vi "Pololu.Mgr - Move to Saved Position.vi"(6 "Ignore Stops":bool, 8 "error in (no error)":errorcluster, 9 "Position Index":i32, 10 "Channel":u8, 11 "PololuCtrl in":refnum<class "PololuCtrl.lvclass">) -> (0 "error out":errorcluster, 1 "Cmd Bytes(Hex)":string, 2 "Position(Deg)":dbl, 3 "PololuCtrl out":refnum<class "PololuCtrl.lvclass">, 4 "Cmd Bytes(Str)":string)   [LabVIEW 2018, in "PololuCtrl.lvclass"]
uses:
  PololuCtrl.lvclass
  PololuCtrl.lvclass/PololuCtrl.ctl
  SubVIs/Pololu.Message Byte Defs.ctl
  Serial Port/Class/SerialPort.lvclass
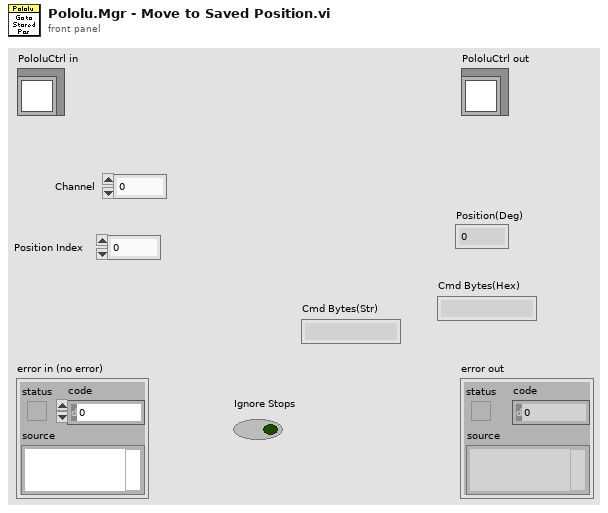
[diagram p1: front panel]
types:
  T1 = typedef "Pololu.Device Config.ctl" = cluster{"Chan":u8, "Accel":u16, "Speed":u16, "Positions":dbl[], "Range Info":T2}
  T2 = typedef "Pololu.Device Range Config.ctl" = cluster{"Min us":dbl, "Max us":dbl, "Min deg":dbl, "Max deg":dbl, "LStopDeg":dbl, "UStopDeg":dbl}
  T3 = cluster{"Channel":u8, "Pos":u16, "Response":u16, "Bytes":u8[], "Query":bool}
  T4 = typedef "Pololu.Message Byte Defs.ctl" = u8
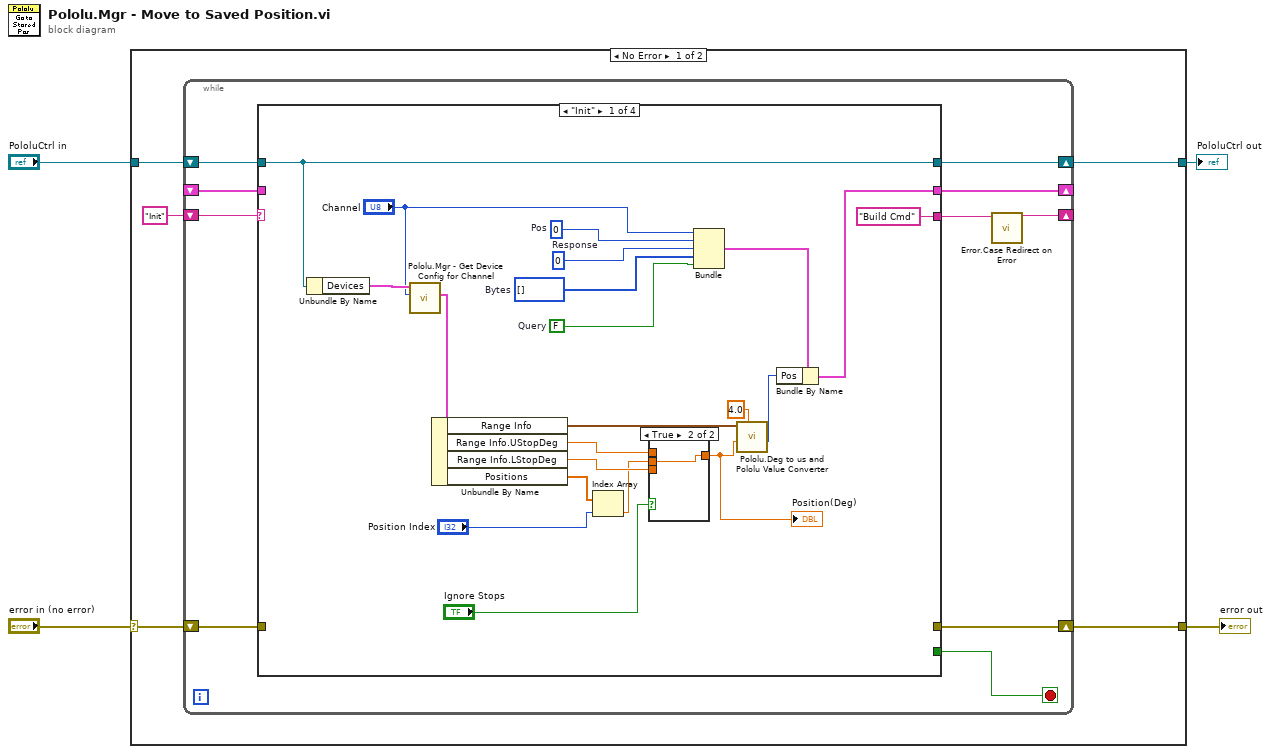
[diagram p0: block diagram]
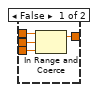
[diagram p2: hidden frame]
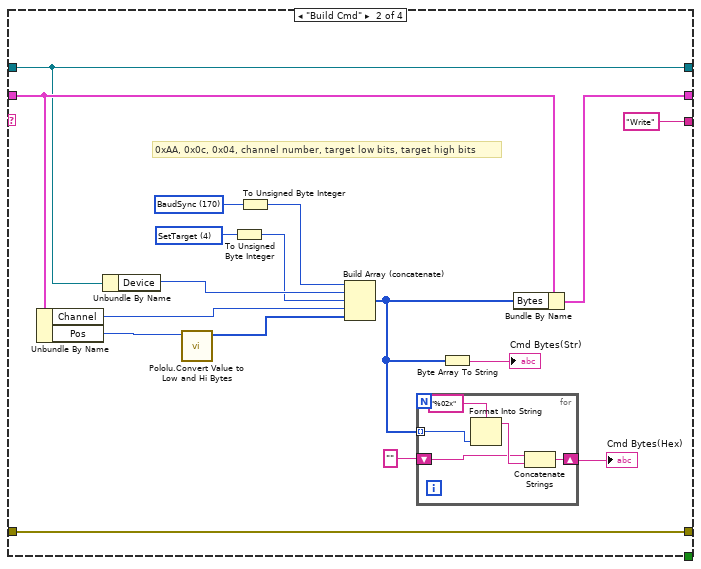
[diagram p3: hidden frame]
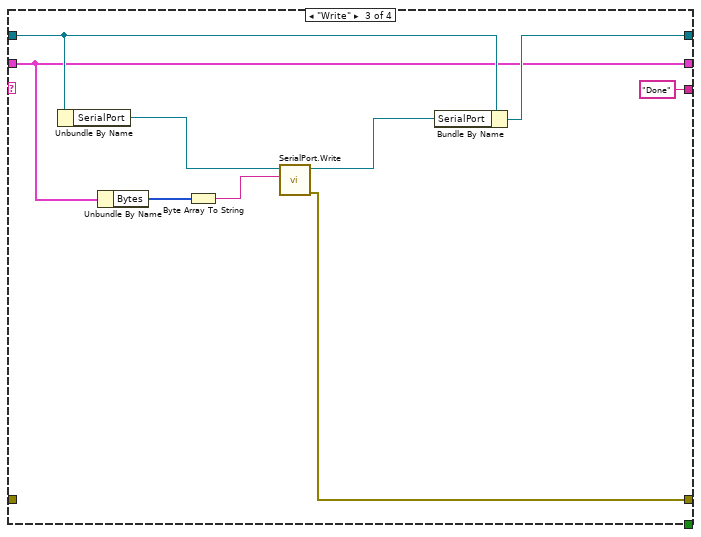
[diagram p4: hidden frame]
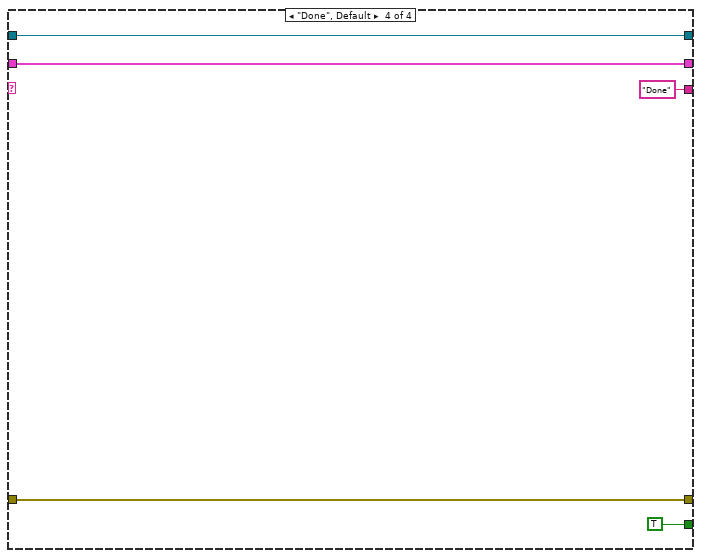
[diagram p5: hidden frame]
diagram:
  n1 = case shown="No Error" "error in (no error)" {
    selector: "error in (no error)" -> [w8 w83]
    tunnel: [w5 w83] -> w3
    tunnel: [w7 w82] -> w1
    tunnel: "PololuCtrl in" -> [w9 w82]
    frame No Error {
      n2 = while {
        shift-right: [w18] -> w7
        shift-left: w9 -> [w19]
        shift-right: [w11] -> w5
        shift-left: w8 -> [w12]
        shift-right: [w15] -> _
        shift-left: "Init" -> [w16]
        shift-right: [w13] -> _
        shift-left: _ -> [w17]
        stop <- w10 stop-if-true
        n3 = case shown="\"Init\"" w16 {
          tunnel: w19 -> [w35 w57 w73 w81]
          tunnel: [w35 w57 w74 w81] -> w18
          tunnel: w17 -> [_ w60 w69 w78]
          tunnel: ["Build Cmd" "Write" "Done" "Done"] -> w14
          tunnel: [w33 w61 w69 w78] -> w13
          tunnel: w12 -> [_ w62 _ w79]
          tunnel: [_ w62 w70 w79] -> w11
          tunnel: [_ _ _ TRUE] -> w10
          frame "Init" {
            w36 = u16 0  # Pos
            w39 = u16 0  # Response
            w37 = FALSE  # Query
            w38 = u8[] []  # Bytes
            n4 = Unbundle By Name(w35) -> ("Devices"=w23:T1[])
            n5 = call "Pololu.Mgr - Get Device Config for Channel.vi"("Channel"="Channel", "Devices"=w23) -> ("Device"=w21:T1)  [unwired: 7 in, 2 out]
            n6 = Unbundle By Name(w21) -> ("Range Info"=w30:T2, "Range Info.UStopDeg"=w32:dbl, "Range Info.LStopDeg"=w31:dbl, "Positions"=w27:dbl[])
            n7 = Index Array(array=w27, index="Position Index") -> (element=w25:dbl)
            n8 = case shown="True" "Ignore Stops" {
              tunnel: w32 -> [w44 _]
              tunnel: w31 -> [w43 _]
              tunnel: w25 -> [w42 w45]
              tunnel: [w41 w45] -> w24
              frame False {
                n9 = In Range and Coerce(upper limit=w44, x=w42, lower limit=w43) -> (coerced(x)=w41:dbl)  [unwired: 1 out]
              }
              frame True {
              }
            }
            "Position(Deg)" <- w24
            n10 = Bundle("Channel"="Channel", "Pos"=w36, "Response"=w39, "Bytes"=w38, "Query"=w37) -> (w34:T3)  [unwired: 1 in]
            n11 = call "Pololu.Deg to us and Pololu Value Converter.vi"("us to Units Mult"=4.0, "Set Pos (Deg)"=w24, "Range Info"=w30) -> ("Cmd units"=w29:u16)  [unwired: 7 in, 1 out]
            n12 = Bundle By Name(cluster=w34, "Pos"=w29) -> (w33:T3)
          }
          frame "Build Cmd" {
            w51 = T4 4 items=["BaudSync"=170, "SetTarget"=4, "Set Speed"=7, "Set Accel"=9, "Get Pos"=16, "Get MovStat"=19, "Get Errors"=33] ("Cmds")
            w52 = T4 170 items=["BaudSync"=170, "SetTarget"=4, "Set Speed"=7, "Set Accel"=9, "Get Pos"=16, "Get MovStat"=19, "Get Errors"=33] ("Cmds")
            # "0xAA, 0x0c, 0x04, channel number, target low bits, target high bits"
            n13 = Unbundle By Name(w60) -> ("Channel"=w59:u8, "Pos"=w58:u16)
            n14 = Unbundle By Name(w57) -> ("Device"=w56:u8)
            n15 = call "Pololu.Convert Value to Low and Hi Bytes.vi"("Value"=w58) -> ("Low_Hi Bytes"=w53:u8[])  [unwired: 10 in]
            n16 = To Unsigned Byte Integer(number=w51) -> (unsigned 8bit integer=w54:T4)
            n17 = To Unsigned Byte Integer(number=w52) -> (unsigned 8bit integer=w55:T4)
            n18 = Build Array (concatenate)(w55, w56, w54, w59, w53) -> (w47:T4[])
            n19 = for {
              tunnel: w47 -> [w67] mode=indexing
              shift-right: [w65] -> w48
              shift-left: "" -> [w63]
              n20 = Format Into String(format string="%02x", w67) -> (resulting string=w64:string)  [unwired: 2 in, 1 out]
              n21 = Concatenate Strings(w63, w64) -> (w65:string)
            }
            "Cmd Bytes(Hex)" <- w48
            n22 = Byte Array To String(unsigned byte array=w47) -> (string=→"Cmd Bytes(Str)":string)
            n23 = Bundle By Name(cluster=w60, "Bytes"=w47) -> (w61:T3)
          }
          frame "Write" {
            n24 = Unbundle By Name(w73) -> ("SerialPort"=w72:refnum<class "SerialPort.lvclass">)
            n25 = Unbundle By Name(w69) -> ("Bytes"=w75:u8[])
            n26 = Byte Array To String(unsigned byte array=w75) -> (string=w68:string)
            n27 = call "SerialPort.Write.vi"("Data"=w68, "SerialPort in"=w72) -> ("error out"=w70:errorcluster, "SerialPort out"=w71:refnum<class "SerialPort.lvclass">)  [unwired: 6 in, 2 out]
            n28 = Bundle By Name(cluster=w73, "SerialPort"=w71) -> (w74:refnum<class "PololuCtrl.lvclass">)
          }
          frame "Done", Default {
          }
        }
        n29 = call "Error.Case Redirect on Error.vi"("Next Case"=w14) -> ("Next Case Out"=w15:string)  [unwired: 10 in]
      }
    }
    frame Error {
    }
  }
  "error out" <- w3
  "PololuCtrl out" <- w1
